vi "Create Message_ValueChangeAndTrigger.vi"(7 "Optional Settings":T1 {"Trigger Channel Refnum" format="%.0x"}, 8 "Error In":errorcluster, 10 "Message Name":string, 11 "Message Group Refnum In":T3=18446744073709551615 format="%.0x") -> (0 "Error Out":errorcluster, 2 "Message Refnum":T3=18446744073709551615 format="%.0x", 3 "Message Group Refnum Out":T3=18446744073709551615 format="%.0x")   [LabVIEW 2020, in "Scripting API.lvlib"]
uses:
  Scripting API.lvlib
  <vilib>/NI VeriStand/Custom Device API/Custom Device Item Ref.ctl
  Examples/Control 3.ctl
  Examples/Control 4.ctl
  <vilib>/NI VeriStand/Custom Device API/Custom Device API.lvlib
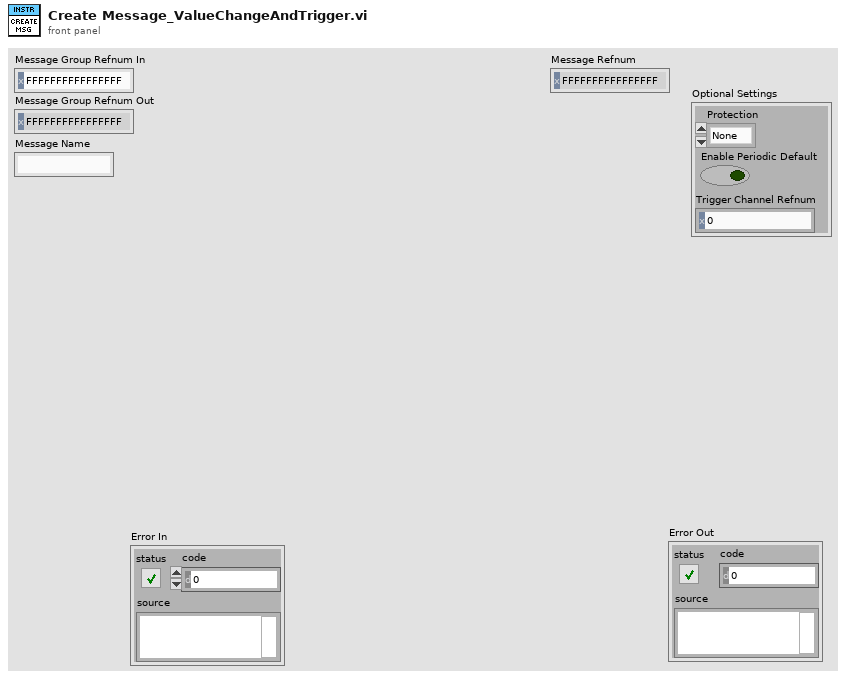
[diagram p1: front panel]
types:
  T1 = typedef "Control 3.ctl" = cluster{"Protection":T2, "Enable Periodic Default":bool, "Trigger Channel Refnum":T3}
  T2 = typedef "Control 4.ctl" = enum16{"None", "CRC-32", "Checksum U8", "Checksum U16", "Checksum U32"}
  T3 = typedef "Custom Device API.lvlib/Custom Device Item Ref.ctl" = u64
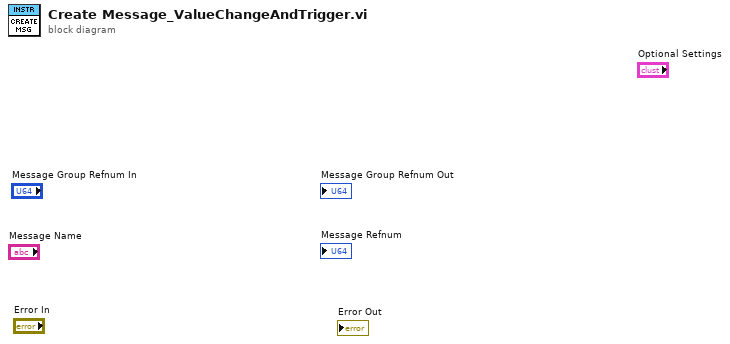
[diagram p0: block diagram]
diagram:
